vi "Place New Grape.vi"(8 "error in (no error)":errorcluster, 9 "Packed refs":T1, 10 "Board Game in":refnum<class "Board Game.lvclass">, 11 "Grape in":refnum<class "Grape.lvclass">) -> (0 "error out":errorcluster, 3 "Grape out":refnum<class "Grape.lvclass">)   [LabVIEW 2021, in "Grape.lvclass"]
uses:
  Grape.lvclass
  C:/Users/poche/Programs/LabVIEW/imposible snake/GameEl_class/GameEl.lvclass
  Board Game_class/Board Game.lvclass
  Application/Packed Refs.ctl
  GameEl_class/private/Enum Direction.ctl
  Imposible_Snake_v2/LVApp/Modules/Sound Manager/Typedefs/Sound Effects.ctl
  GameEl_class/GameEl.lvclass/GameEl.ctl
  Grape.lvclass/Grape.ctl
  GameEl_class/GameEl.lvclass
  Imposible_Snake_v2/LVApp/Modules/Sound Manager/Sound Manager.lvlib
  Application/Game.lvclass
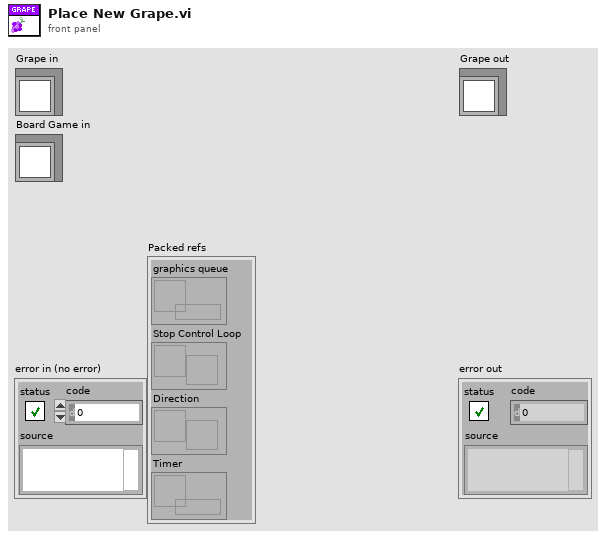
[diagram p1: front panel]
types:
  T1 = typedef "Game.lvclass/Packed Refs.ctl" = cluster{"graphics queue":refnum<queue>, "Stop Control Loop":refnum<user-event>, "Direction":refnum<notifier>, "Timer":refnum<data-value>}
  T2 = typedef "Sound Manager.lvlib/Sound Effects.ctl" = enum16{"Bomb In", "Bomb Out", "Bomb Touched", "Game Over", "Victory", "Eat", "10 Fruits", "Eat2", "Eat3", "Eat4", "MaxShield", "Shield", "10p", "Grape In", "Grape Out", "20p", "30p", "40p", "50p", "60p", "70p", "80p", "90p", "100p", "All shields cracked", "Mouse In", "Mouse Out", "Mouse Eaten", "Grape Eaten", "States Recover", "Broken Shield", "Bonus", "Happy Time", "explode", "Game over musica", "Back Music", "Shield Catch", "Evil lough", "Cricket In", "Cricket eaten", "Lets Go", "Jump1", "Jump2", "Jump3", "Unstoppable", "Troll Music", "winner", "menu"}
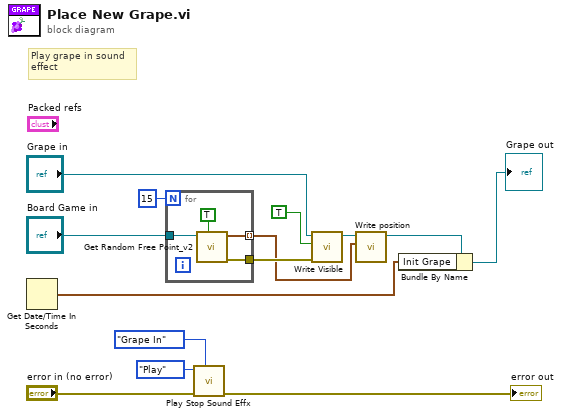
[diagram p0: block diagram]
diagram:
  # "Play grape in sound\neffect"
  n1 = Get Date/Time In Seconds() -> (seconds since 1Jan1904=w12:timestamp)
  n2 = for {
    N: 15 -> [_]
    tunnel: "Board Game in" -> [w18]
    tunnel: [w17] -> w7
    tunnel: [w16] -> w5 mode=indexing
    n3 = call "Get Random Free Point_v2.vi"("Safe Area?"=TRUE, "Board Game in"=w18) -> ("error out"=w17:errorcluster, "Position"=w16:cluster{"X":dbl, "Y":dbl})  [unwired: 8 in]
  }
  n4 = call "Play Stop Sound Effx.vi"("Sound Effect"=Sound_Effects."Grape In", "Error In"="error in (no error)", "Function"=enum16{"Play", "Stop"}."Play") -> ("error in (no error)"=→"error out":errorcluster)  [unwired: 8 in]
  n5 = call "Write Visible.vi"("error in (no error)"=w7, "Visible"=TRUE, "GameEl in"="Grape in") -> ("GameEl out"=w11:refnum<class "Grape.lvclass">)  [unwired: 7 in, 1 out]
  n6 = call "Write position.vi"("position"=w5, "GameEl in"=w11) -> ("GameEl out"=w10:refnum<class "Grape.lvclass">)  [unwired: 8 in, 1 out]
  n7 = Bundle By Name(cluster=w10, "Init Grape"=w12) -> (→"Grape out":refnum<class "Grape.lvclass">)
